vi "Modbus.DataNotifier.vi"(7 "OP":enum16{"Read", "Write"}(ring), 11 "notifier IN":refnum<notifier>) -> (3 "notifier OUT":refnum<notifier>)   [LabVIEW 2019, in "Modbus.lvlib"]
uses:
  Modbus.lvlib
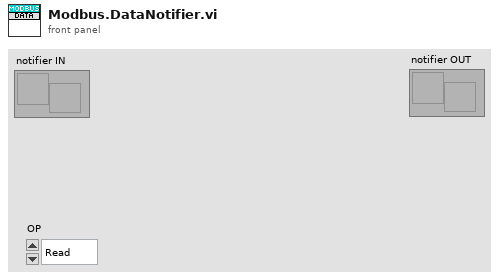
[diagram p1: front panel]
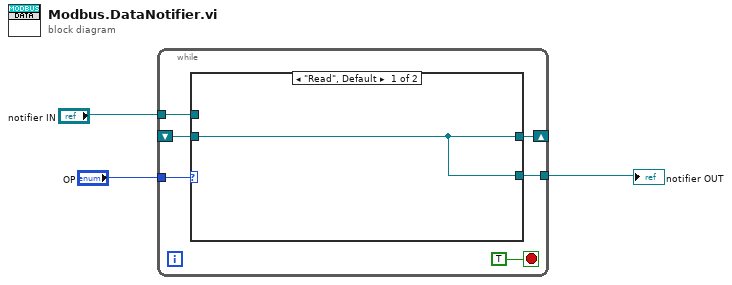
[diagram p0: block diagram]
diagram:
  n1 = while {
    tunnel: "OP" -> [w8]
    tunnel: "notifier IN" -> [w6]
    shift-right: [w7] -> _
    shift-left: _ -> [w5]
    tunnel: [w4] -> w1
    stop <- TRUE stop-if-true
    n2 = case shown="\"Read\", Default" w8 {
      tunnel: [w10 w11] -> w7
      tunnel: w6 -> [_ w11]
      tunnel: w5 -> [w10 _]
      tunnel: [w10 _] -> w4
      frame "Read", Default {
      }
      frame "Write" {
      }
    }
  }
  "notifier OUT" <- w1
